vi "uwave_scanner_usb4000.vi"() -> ()   [LabVIEW 2018]
uses:
  <vilib>/Utility/file.llb/Write Delimited Spreadsheet (DBL).vi
  <instrlib>/Stanford Research SG380 Series/Stanford Research SG380 Series.lvlib
panel:
  out "Waveform Chart":dbl[](graph)
  in  "Background":bool
  in  "Width":i32(slide) scale=0.0..500.0
  in  "Start":i32(slide) scale=0.0..3500.0
  out "WL Values":dbl[](array[numeric])
  out "Length":i32
  out "XY Graph":T1(graph)
  out "Number of Spectrometers":i32
  in  "microwaves":bool
  out "Detuning":dbl
  out "Ch1":cluster{dbl[], dbl[]}(graph)
  in  "Step Delta":dbl=50.0 format="%#_13g"
  out "error out":errorcluster
  out "f":dbl format="%#.10g"
  in  "stop":bool
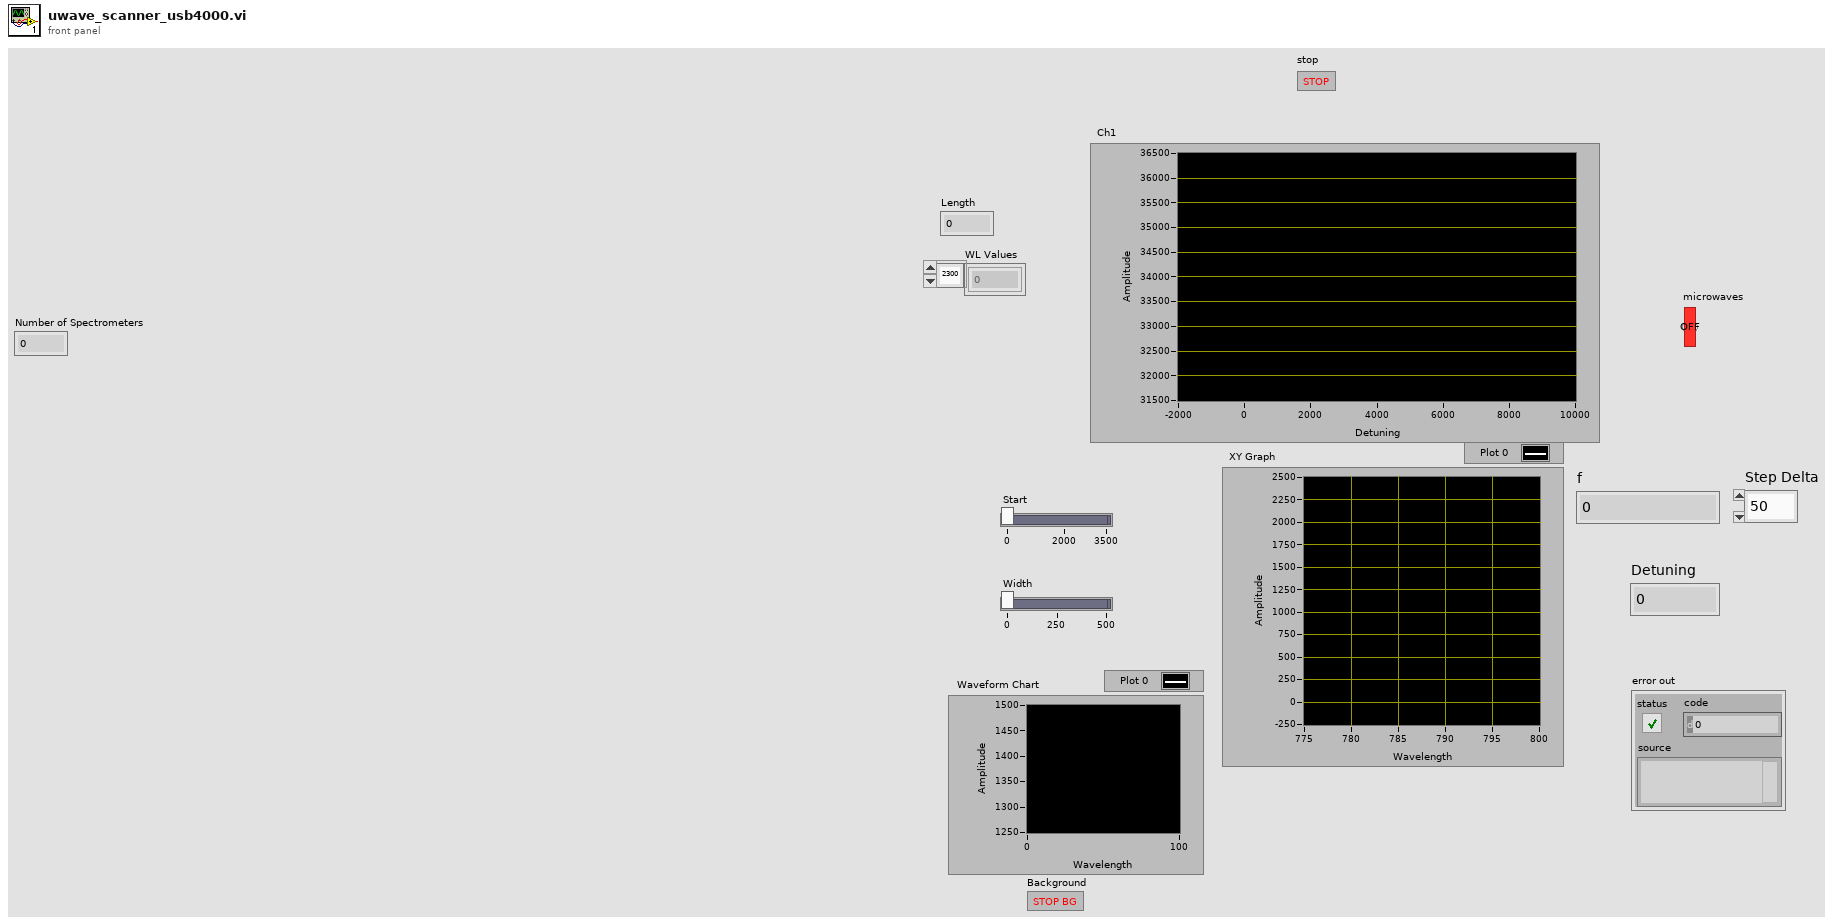
[diagram p1: front panel]
types:
  T1 = cluster{"Spectrum Values":dbl[], "Spectrum Values":dbl[]}
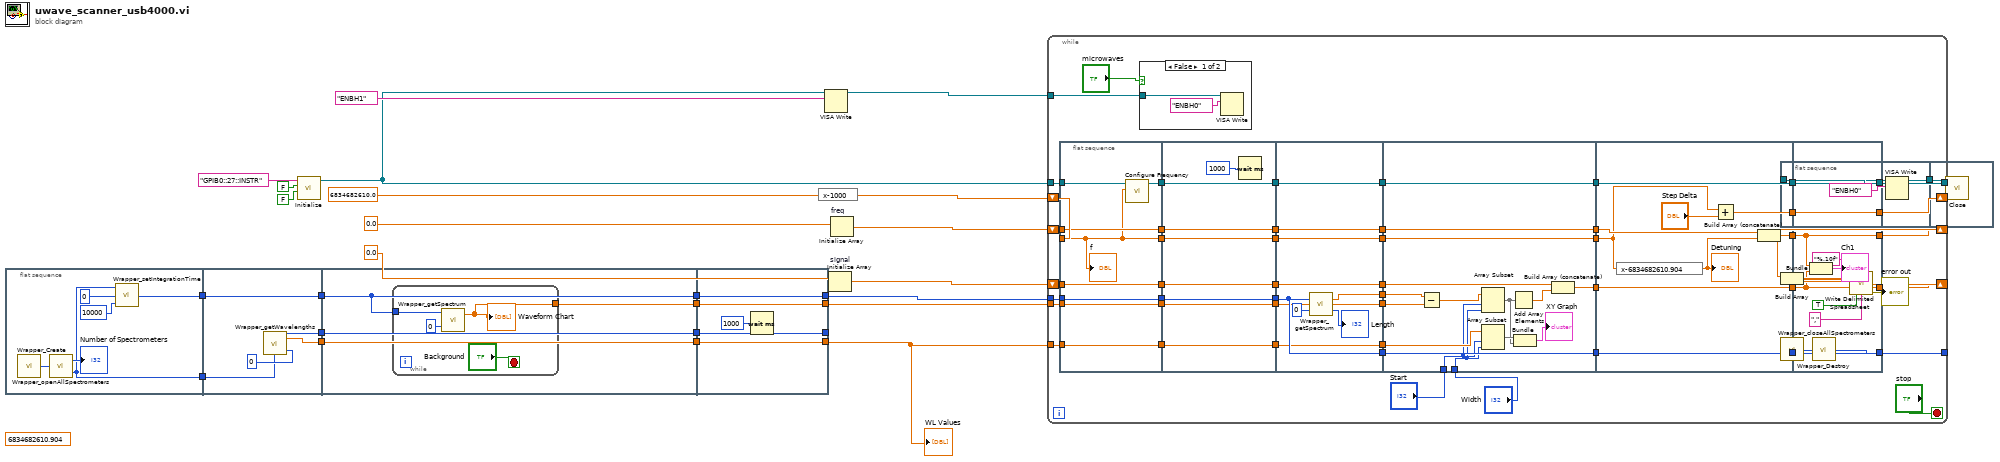
[diagram p0: block diagram]
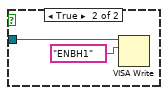
[diagram p2: hidden frame]
diagram:
  (unwired) 6834682610.904
  n1 = flat-sequence {
    tunnel: [w37] -> w12
    tunnel: [w36] -> w9
    tunnel: w12 -> [w43]
    tunnel: w9 -> [w42]
    tunnel: [w44] -> w8
    tunnel: [w43] -> w7
    tunnel: [w42] -> w6
    tunnel: w8 -> [w49]
    tunnel: w7 -> [w48]
    tunnel: w6 -> [w47]
    tunnel: [w49] -> w4
    tunnel: [w48] -> w3
    tunnel: [w47] -> w2
    tunnel: [w46] -> w1
    tunnel: [w55] -> w5
    tunnel: [w56] -> w10
    tunnel: [w57] -> _
    tunnel: [w58] -> w13
    tunnel: w4 -> [w58]
    tunnel: w3 -> [w57]
    tunnel: w2 -> [w56]
    tunnel: w1 -> [w55]
    frame #0 {
      n2 = call "Wrapper_Create.vi"() -> ("Wrapper"=w40:u64)
      n3 = call "Wrapper_openAllSpectrometers.vi"("Wrapper In"=w40) -> ("Number of Spectrometers"=→"Number of Spectrometers":i32, "Wrapper Out"=w37:u64)
      n4 = call "Wrapper_setIntegrationTime.vi"("Integration Time"=10000, "Index"=0, "Wrapper In"=w37) -> ("Wrapper Out"=w36:u64)
    }
    frame #1 {
      n5 = call "Wrapper_getWavelengths.vi"("Index"=0, "Wrapper"=w43) -> ("WL Values"=w44:dbl[])  [unwired: 1 out]
    }
    frame #2 {
      n6 = while {
        tunnel: w47 -> [w52]
        tunnel: [w50] -> w46
        stop <- "Background" stop-if-true
        n7 = call "Wrapper_getSpectrum.vi"("Index"=0, "Wrapper"=w52) -> ("Spectrum Values"=w50:dbl[])  [unwired: 1 out]
        "Waveform Chart" <- w50
      }
    }
    frame #3 {
      n8 = Wait (ms)(milliseconds to wait=u32 1000) -> ()  [unwired: 1 out]
    }
  }
  n9 = call <instrlib>:"Initialize.vi"("Reset (True)"=FALSE, "ID Query (True)"=FALSE, "VISA resource name"="GPIB0::27::INSTR") -> ("VISA resource name out"=w22:refnum<visa-resource-name>)  [unwired: 7 in, 1 out]
  n10 = expression code="x-1000"(6834682610.0) -> (w17:dbl)
  n11 = VISA Write(VISA resource name=w22, write buffer="ENBH1" ("data")) -> (VISA resource name out=w18:refnum<visa-resource-name>)  [unwired: 1 in, 2 out]
  n12 = Initialize Array "signal"(0.0 ("element")) -> (w16:dbl[])  [unwired: 1 in]
  n13 = Initialize Array "freq"(0.0 ("element")) -> (w32:dbl[])  [unwired: 1 in]
  n14 = while {
    shift-right: [w87] -> w29
    shift-left: w32 -> [w106]
    tunnel: w22 -> [w105]
    tunnel: [w103] -> w21
    tunnel: w18 -> [w95]
    shift-right: [w86] -> w15
    shift-left: w16 -> [w90]
    tunnel: w13 -> [w75]
    tunnel: w10 -> [w72]
    tunnel: [w71] -> w11
    shift-right: [w66] -> _
    shift-left: w17 -> [w94]
    tunnel: w5 -> [w59]
    stop <- "stop" stop-if-true
    n15 = flat-sequence {
      tunnel: [w119] -> w101
      tunnel: w106 -> [w119]
      tunnel: w105 -> [w118]
      tunnel: [w117] -> w100
      tunnel: w94 -> [w115]
      tunnel: [w115] -> w92
      tunnel: [w116] -> w91
      tunnel: w90 -> [w116]
      tunnel: [w114] -> w76
      tunnel: w75 -> [w114]
      tunnel: [w113] -> w73
      tunnel: w72 -> [w113]
      tunnel: [w112] -> w60
      tunnel: w59 -> [w112]
      tunnel: w101 -> [w127]
      tunnel: [w127] -> w85
      tunnel: w100 -> [w126]
      tunnel: [w126] -> w83
      tunnel: [w124] -> w81
      tunnel: w92 -> [w124]
      tunnel: [w123] -> w79
      tunnel: w91 -> [w123]
      tunnel: [w122] -> w77
      tunnel: w76 -> [w122]
      tunnel: [w121] -> w74
      tunnel: w73 -> [w121]
      tunnel: [w120] -> w61
      tunnel: w60 -> [w120]
      tunnel: w85 -> [w137]
      tunnel: [w137] -> w84
      tunnel: w83 -> [w136]
      tunnel: [w136] -> w82
      tunnel: w81 -> [w135]
      tunnel: [w135] -> w80
      tunnel: w79 -> [w134]
      tunnel: [w134] -> w78
      tunnel: w77 -> [w129]
      tunnel: w74 -> [w131]
      tunnel: [w131] -> w68
      tunnel: [w130] -> w67
      tunnel: [w129] -> w65
      tunnel: [w128] -> w62
      tunnel: w61 -> [w128]
      tunnel: [w153] -> w104
      tunnel: w84 -> [w153]
      tunnel: [w152] -> w102
      tunnel: w82 -> [w152]
      tunnel: [w151] -> w93
      tunnel: w80 -> [w151]
      tunnel: w78 -> [w150]
      tunnel: [w148] -> w89
      tunnel: [w147] -> w69
      tunnel: w68 -> [w147]
      tunnel: w67 -> [w140]
      tunnel: w65 -> [w146]
      tunnel: "Start" -> [w142]
      tunnel: "Width" -> [w141]
      tunnel: w62 -> [w138]
      tunnel: w104 -> [w160]
      tunnel: w102 -> [w158]
      tunnel: [w161] -> w99
      tunnel: [w159] -> w98
      tunnel: [w158] -> w97
      tunnel: w93 -> [w154]
      tunnel: w89 -> [w157]
      tunnel: [w157] -> w88
      tunnel: [w155] -> w70
      tunnel: w69 -> [w155]
      tunnel: [w168] -> w103
      tunnel: w99 -> [w163]
      tunnel: w98 -> [w166]
      tunnel: w97 -> [w168]
      tunnel: w88 -> [w165]
      tunnel: [w166] -> w87
      tunnel: [w165] -> w86
      tunnel: [w164] -> w71
      tunnel: w70 -> [w164]
      tunnel: [w163] -> w66
      frame #0 {
        n16 = call <instrlib>:"Configure Frequency.vi"("Carrier Frequency (1E+7 Hz)"=w115, "VISA resource name"=w118) -> ("VISA resource name out"=w117:refnum<visa-resource-name>)  [unwired: 8 in, 1 out]
        "f" <- w115
      }
      frame #1 {
        n17 = Wait (ms)(milliseconds to wait=u32 1000) -> ()  [unwired: 1 out]
      }
      frame #2 {
        n18 = call "Wrapper_getSpectrum.vi"("Index"=0, "Wrapper"=w131) -> ("Length"=→"Length":i32, "Spectrum Values"=w130:dbl[])
      }
      frame #3 {
        n19 = Subtract(x=w140, y=w138) -> (x-y=w139:dbl[])
        n20 = Array Subset(array=w139, index=w142, length=w141) -> (w143:dbl[])
        n21 = Array Subset(array=w146, index=w142, length=w141) -> (w144:dbl[])
        n22 = Add Array Elements(numeric array=w143) -> (sum=w149:dbl)
        n23 = Bundle(w144, w143) -> (→"XY Graph":cluster{dbl[], dbl[]})  [unwired: 1 in]
        n24 = Build Array (concatenate)(w150, w149) -> (w148:dbl[])
      }
      frame #4 {
        n25 = expression code="x-6834682610.904"(w154) -> (w156:dbl)
        "Detuning" <- w156
        n26 = Add(x=w154, y="Step Delta") -> (x+y=w161:dbl)
        n27 = Build Array (concatenate)(w160, w156) -> (w159:dbl[])
      }
      frame #5 {
        n28 = Bundle(w166, w165) -> (→"Ch1":cluster{dbl[], dbl[]})  [unwired: 1 in]
      }
    }
    n29 = case shown="False" "microwaves" {
      tunnel: w95 -> [w108 w110]
      frame False {
        n30 = VISA Write(VISA resource name=w108, write buffer="ENBH0" ("data")) -> ()  [unwired: 1 in, 3 out]
      }
      frame True {
        n31 = VISA Write(VISA resource name=w110, write buffer="ENBH1" ("data")) -> ()  [unwired: 1 in, 3 out]
      }
    }
  }
  n32 = flat-sequence {
    tunnel: w21 -> [w170]
    tunnel: [w169] -> w20
    tunnel: w20 -> [w172]
    frame #0 {
      n33 = VISA Write(VISA resource name=w170, write buffer="ENBH0" ("data")) -> (VISA resource name out=w169:refnum<visa-resource-name>)  [unwired: 1 in, 2 out]
    }
    frame #1 {
      n34 = call <instrlib>:"Close.vi"("VISA resource name"=w172) -> ()  [unwired: 10 in, 1 out]
    }
  }
  n35 = Build Array(w29, w15) -> (w28:dbl[][])
  n36 = call "Wrapper_closeAllSpectrometers.vi"("Wrapper In"=w11) -> ("Wrapper Out"=w14:u64)
  n37 = call "Wrapper_Destroy.vi"("Wrapper"=w14) -> ()
  n38 = call-poly <vilib>:"Write Delimited Spreadsheet.vi"("format (%.3f)"="%.10f", "2D data"=w28, "transpose? (no:F)"=TRUE, "delimiter (\\t)"="," ("delimiter (\\t)")) -> ("error out"=→"error out":errorcluster)  [unwired: 10 in, 1 out]
  "WL Values" <- w13
